vi "varXNode_Mutate_1_0_0_6.vi"(8 "error in (no error)":errorcluster, 9 "Replies in":string[](array[string]), 10 "Version":T1, 11 "Old State":variant) -> (0 "error out":errorcluster, 1 "Replies out":string[](array[string]), 2 "Version Out":T1, 3 "New State":variant)   [LabVIEW 2017, in "varXNode.xnode"]
uses:
  <vilib>/variable/varXNode.llb/varXNode.xnode
  <vilib>/XNodeSupport/XNodeVersion.ctl
  <vilib>/XNodeSupport/XNodeUShort.ctl
  <vilib>/variable/varXNode.llb/varXNode_old_1_0_0_4.ctl
  <vilib>/variable/varXNode.llb/varXNode_old_1_0_0_6.ctl
  <vilib>/variable/Type Descriptor.ctl
  <vilib>/XNodeSupport/NI_XNodeSupport.lvlib
  <vilib>/variable/NI_Variable.lvlib
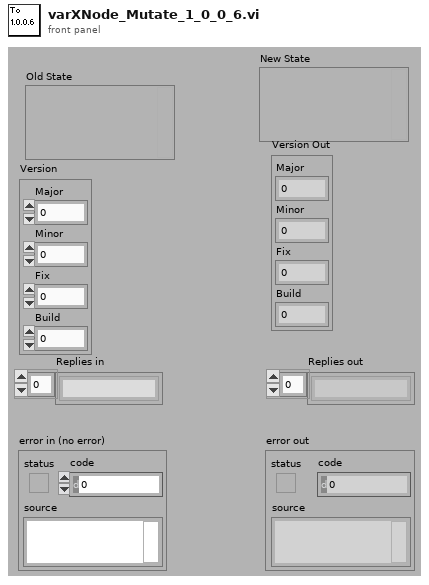
[diagram p1: front panel]
types:
  T1 = typedef "NI_XNodeSupport.lvlib/XNodeVersion.ctl" = cluster{"Major":T2, "Minor":T2, "Fix":T2, "Build":T2}
  T2 = typedef "NI_XNodeSupport.lvlib/XNodeUShort.ctl" = u16
  T3 = typedef "varXNode.xnode/varXNode_old_1_0_0_6.ctl" = cluster{"Write":bool, "ShowTimestamp":bool, "CachedName":string, "CachedTypeDesc":T4, "CachedFeaturePacks":string[], "Custom Rule":string, "ProjectPath":string, "Bad Code":bool, "ContextName":string}
  T4 = typedef "NI_Variable.lvlib/Type Descriptor.ctl" = cluster{"Variant":variant}
  T5 = typedef "varXNode.xnode/varXNode_old_1_0_0_4.ctl" = cluster{"Write":bool, "ShowTimestamp":bool, "CachedName":string, "CachedTypeDesc":i16[], "CachedFeaturePacks":string[], "Custom Rule":string, "ProjectPath":string, "Bad Code":bool, "ContextName":string}
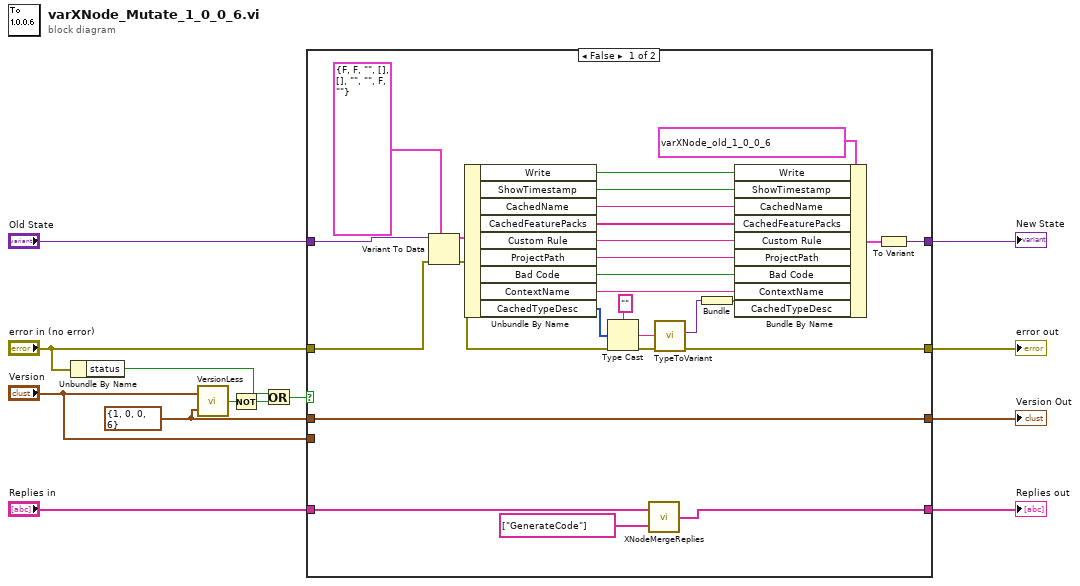
[diagram p0: block diagram]
diagram:
  w12 = T1 {"Major"=1, "Minor"=0, "Fix"=0, "Build"=6} ("y")
  n1 = Unbundle By Name("error in (no error)") -> ("status"=w4:bool)
  n2 = call <vilib>:"VersionLess.vi"("y"=w12, "x"="Version") -> ("x < y?"=w13:bool)
  n3 = Not(x=w13) -> (.not. x?=w3:bool)
  n4 = Or(x=w4, y=w3) -> (x .or. y?=w6:bool)
  n5 = case shown="False" w6 {
    tunnel: w12 -> [w39 _]
    tunnel: [w28 w43] -> w11
    tunnel: "Old State" -> [w38 w43]
    tunnel: [w39 w42] -> w9
    tunnel: "Version" -> [_ w42]
    tunnel: [w20 w41] -> w7
    tunnel: "error in (no error)" -> [w16 w41]
    tunnel: [w18 w40] -> w2
    tunnel: "Replies in" -> [w19 w40]
    frame False {
      n6 = Variant To Data(error in=w16, type=T5 {"Write"=FALSE, "ShowTimestamp"=FALSE, "CachedName"="", "CachedTypeDesc"=[], "CachedFeaturePacks"=[], "Custom Rule"="", "ProjectPath"="", "Bad Code"=FALSE, "ContextName"=""} ("State"), Variant=w38) -> (data=w37:T5, error out=w15:errorcluster)
      n7 = Unbundle By Name(w37) -> ("Write"=w36:bool, "ShowTimestamp"=w35:bool, "CachedName"=w34:string, "CachedFeaturePacks"=w33:string[], "Custom Rule"=w32:string, "ProjectPath"=w31:string, "Bad Code"=w30:bool, "ContextName"=w29:string, "CachedTypeDesc"=w24:i16[])
      n8 = Type Cast(type="", x=w24) -> (*(type *) &x=w25:string)
      n9 = call <vilib>:"XNodeMergeReplies.vi"("New Replies"=string[] ["GenerateCode"], "Old Replies"=w19) -> ("Merged Replies"=w18:string[])
      n10 = call <vilib>:"TypeToVariant.vi"("error in (no error)"=w15, "typeCode"=w25) -> ("error out"=w20:errorcluster, "Variant"=w22:variant)  [unwired: 4 in]
      n11 = Bundle("Variant"=w22) -> (w21:cluster{"Variant":variant})  [unwired: 1 in]
      n12 = Bundle By Name(cluster=T3 {"Write"=FALSE, "ShowTimestamp"=FALSE, "CachedName"="", "CachedTypeDesc"={"Variant"=variant}, "CachedFeaturePacks"=[], "Custom Rule"="", "ProjectPath"="", "Bad Code"=FALSE, "ContextName"=""} ("State"), "Write"=w36, "ShowTimestamp"=w35, "CachedName"=w34, "CachedFeaturePacks"=w33, "Custom Rule"=w32, "ProjectPath"=w31, "Bad Code"=w30, "ContextName"=w29, "CachedTypeDesc"=w21) -> (w27:T3)
      n13 = To Variant(anything=w27) -> (Variant=w28:variant)
    }
    frame True {
      # "Either there was an error in,\nor the version is not less than 1.0.0.6.\nPass input values out."
    }
  }
  "New State" <- w11
  "Version Out" <- w9
  "error out" <- w7
  "Replies out" <- w2
